vi "ArthOps.vi"() -> ()   [LabVIEW 2026]
panel:
  out "x/y":dbl
  out "x+y":dbl
  out "x*y":dbl
  out "x-1":dbl
  out "x*2^n":dbl
  in  "x":dbl
  in  "y":dbl
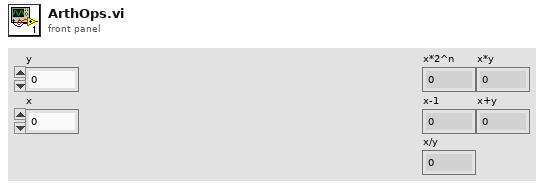
[diagram p1: front panel]
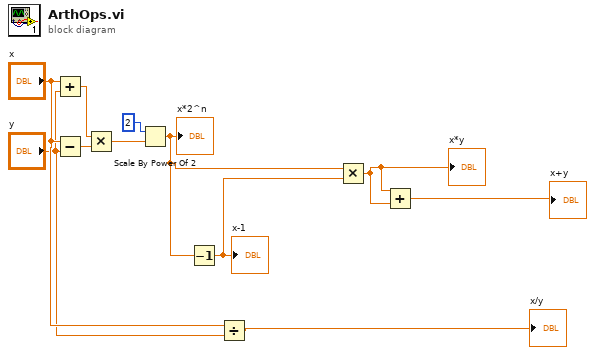
[diagram p0: block diagram]
diagram:
  n1 = Add(x="x", y="y") -> (x+y=w11:dbl)
  n2 = Subtract(x="x", y="y") -> (x-y=w10:dbl)
  n3 = Multiply(x=w11, y=w10) -> (x*y=w9:dbl)
  n4 = Scale By Power Of 2(n=i16 2, x=w9) -> (x*2^n=w7:dbl)
  "x*2^n" <- w7
  n5 = Decrement(x=w7) -> (x-1=w6:dbl)
  "x-1" <- w6
  n6 = Divide(x="x", y="y") -> (x/y=→"x/y":dbl)
  n7 = Multiply(x=w7, y=w6) -> (x*y=w5:dbl)
  "x*y" <- w5
  n8 = Add(x=w5, y=w5) -> (x+y=→"x+y":dbl)
